vi "Load.vi"(8 "Trained?":bool, 9 "Trained Path":path, 10 "Left Hem Path":path, 11 "Right Hem Path":path) -> (3 "Cerebellum out":refnum<class "Cerebellum.lvclass">)   [LabVIEW 2013, in "Cerebellum.lvclass"]
uses:
  Cerebellum.lvclass
  AER/AER.lvclass
  Cerebellum.lvclass/Cerebellum.ctl
  <vilib>/Utility/xml.llb/Read From XML File(string).vi
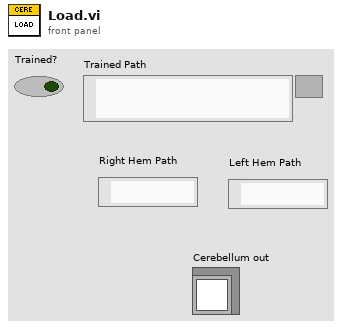
[diagram p1: front panel]
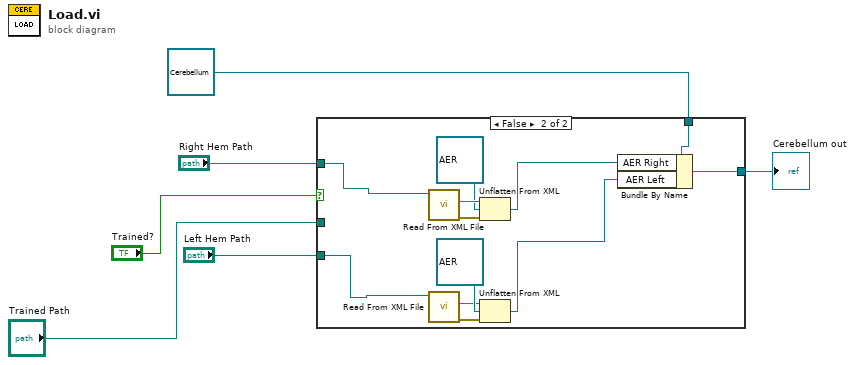
[diagram p0: block diagram]
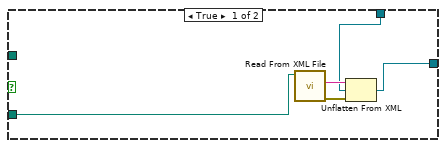
[diagram p2: hidden frame]
diagram:
  n1 = case shown="False" "Trained?" {
    tunnel: refnum<class "Cerebellum.lvclass"> refnum ("Cerebellum in") -> [w9 w23]
    tunnel: [w8 w22] -> w5
    tunnel: "Trained Path" -> [w7 _]
    tunnel: "Right Hem Path" -> [_ w13]
    tunnel: "Left Hem Path" -> [_ w12]
    frame True {
      n2 = call-poly <vilib>:"Read From XML File.vi"("XML File Path"=w7) -> ("error out"=w11:errorcluster, "XML Elements"=w10:string)  [unwired: 8 in, 1 out]
      n3 = Unflatten From XML(xml string=w10, type=w9, error in (no error)=w11) -> (value=w8:refnum<class "Cerebellum.lvclass">)  [unwired: 1 out]
    }
    frame False {
      n4 = call-poly <vilib>:"Read From XML File.vi"("XML File Path"=w13) -> ("error out"=w20:errorcluster, "XML Elements"=w21:string)  [unwired: 8 in, 1 out]
      n5 = call-poly <vilib>:"Read From XML File.vi"("XML File Path"=w12) -> ("error out"=w17:errorcluster, "XML Elements"=w16:string)  [unwired: 8 in, 1 out]
      n6 = Unflatten From XML(xml string=w21, type=refnum<class "AER.lvclass"> refnum ("AER.lvclass"), error in (no error)=w20) -> (value=w15:refnum<class "AER.lvclass">)  [unwired: 1 out]
      n7 = Unflatten From XML(xml string=w16, type=refnum<class "AER.lvclass"> refnum ("AER.lvclass"), error in (no error)=w17) -> (value=w14:refnum<class "AER.lvclass">)  [unwired: 1 out]
      n8 = Bundle By Name(cluster=w23, "AER Right"=w15, "AER Left"=w14) -> (w22:refnum<class "Cerebellum.lvclass">)
    }
  }
  "Cerebellum out" <- w5
